vi "TSPopup.Monitor Events.vi"(9 "Debug":bool, 10 "Unregister\nAll Events":bool=TRUE, 11 "TSPopup":refnum<class "TSPopup.lvclass">) -> ()   [LabVIEW 2016, in "TSPopup.lvlib" / "TSPopup.lvclass"]
doc: "Background process that monitors appropriate events when a popup is shown. Sends feedback when popup is complete.\n\nType Sensitive Popup \nCopyright © 2007, J. David Saunders\nAll rights reserved."
uses:
  <userlib>/TSPopup/TSPopup.lvclass
  <userlib>/TSPopup/TSPopup.lvclass/TSPopup.ctl
  <userlib>/TSPopup/Private/TSPopup.Event Enum.ctl
  <userlib>/TSPopup/Private/TSPopup.Popup Results.ctl
  <vilib>/event_ctls.llb/eventvkey.ctl
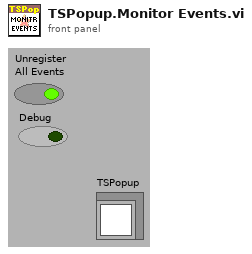
[diagram p1: front panel]
types:
  T1 = enum32{"Invalid", "Standard", "Closed", "Hidden", "Minimized", "Maximized"}
  T2 = typedef "TSPopup.lvlib/TSPopup.lvclass/TSPopup.Event Enum.ctl" = enum16{"Nothing", "Enter Key Accept", "Escape Key Cancel", "Mouse Outside Accept", "Mouse Outside Cancel", "Mouse Move Accept", "Mouse Move Cancel", "Mouse Leave Cancel", "Value Change Accept", "Lose Focus Cancel", "Cancel Button", "Accept Button"}
  T3 = typedef "TSPopup.lvlib/TSPopup.lvclass/TSPopup.Popup Results.ctl" = cluster{"Valid?":bool, "Value Changed?":bool, "Popup Value":variant, "Call Data":variant}
  T4 = typedef "eventvkey.ctl" = enum16{"ASCII", "Enter", "Return", "Shift", "Ctrl", "Alt", "Cmd", "Opt", "Caps", "NumLock", "Clear", "Break", "Up", "Down", "Left", "Right", "Insert", "Delete", "Home", "End", "PageUp", "PageDown", "Escape", "Help", "Pause", "ScrollLock", "F1", "F2", "F3", "F4", "F5", "F6", "F7", "F8", "F9", "F10", "F11", "F12", "F13", "F14", "F15", "F16", "F17", "F18", "F19", "F20", "F21", "F22", "F23", "F24", "Play", "VolumeUp", "VolumeDown", "Mute", "Two Byte Char"}
  T5 = enum32{"Bad", "Idle", "Run top level", "Running"}
  T6 = typedef "TSPopup.lvlib/TSPopup.lvclass/TSPopup.Popup Call Parameters.ctl" = cluster{"Prop Type":T7, "Initial Value":variant, "Caption Strings":string[], "Ring Strings":string[], "Cell Rect":cluster{"left":i16, "top":i16, "right":i16, "bottom":i16}, "Mouse Coords":cluster{"x":i16, "y":i16}, "Call Data":variant}
  T7 = typedef "TSPopup.lvlib/TSPopup.lvclass/TSPopup.Data Type.ctl" = enum16{"Unkown", "NO POPUP", "String", "Integer", "Float", "Color", "Boolean", "Ring", "Captioned String", "Captioned Integer", "Button Color", "2 Int Cluster", "4 Int Cluster", "check"}
  T8 = typedef "LVPoint32TypeDef.ctl" = cluster{"Horizontal":i32, "Vertical":i32}
  T9 = typedef "LVRectTypeDef.ctl" = cluster{"Left":i16, "Top":i16, "Right":i16, "Bottom":i16}
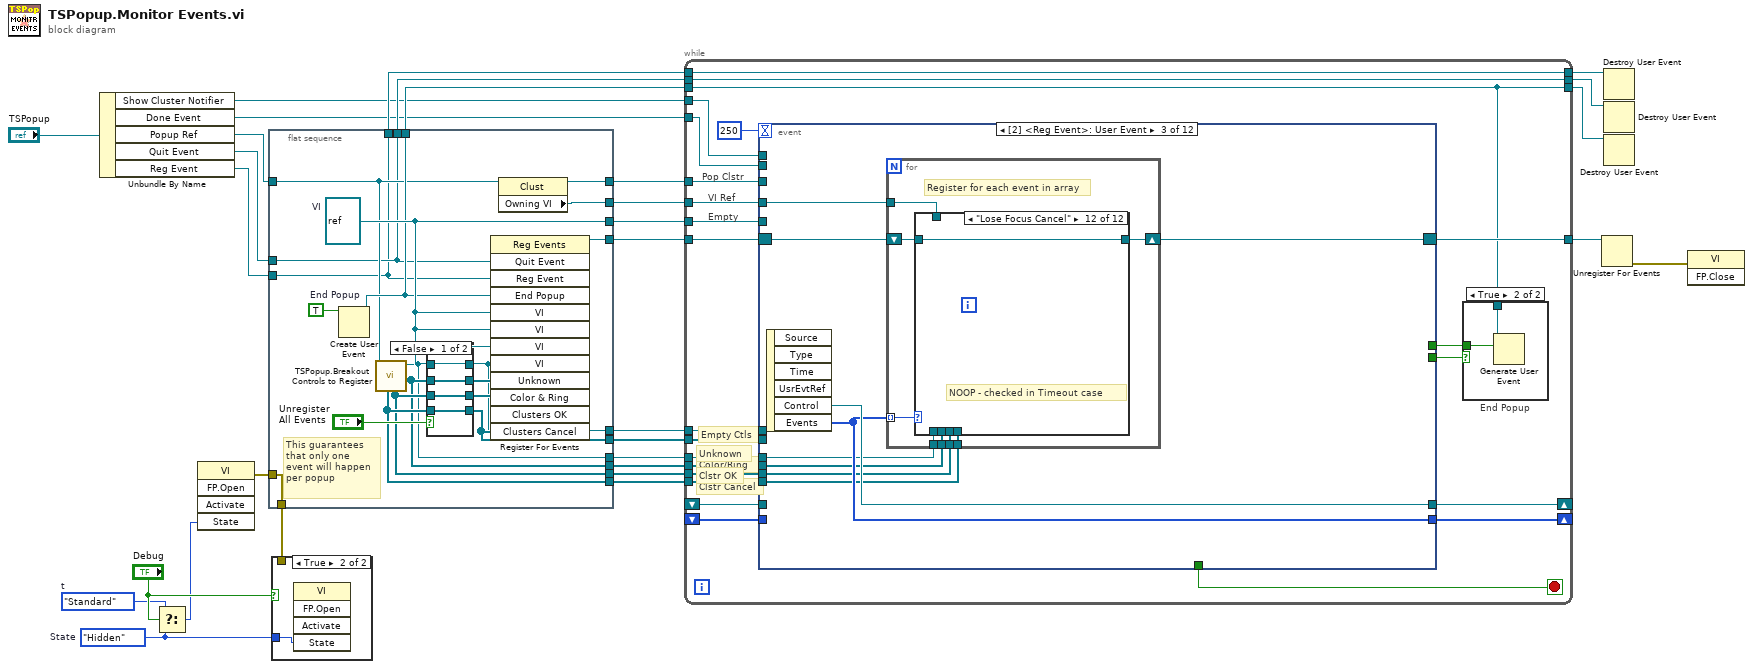
[diagram p0: block diagram]
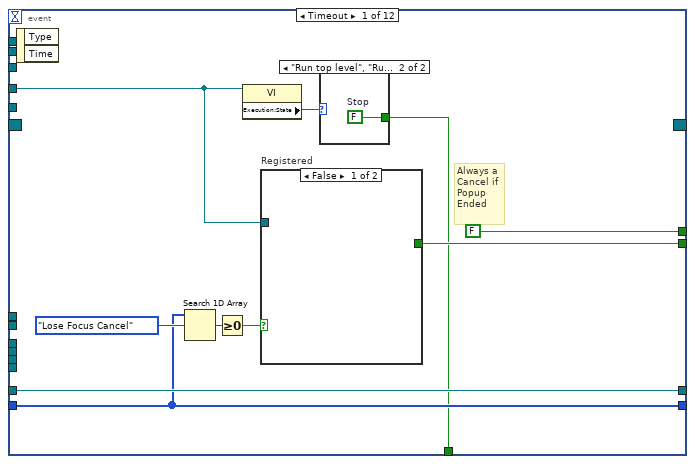
[diagram p5: hidden frame]
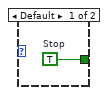
[diagram p6: hidden frame]
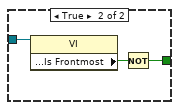
[diagram p7: hidden frame]
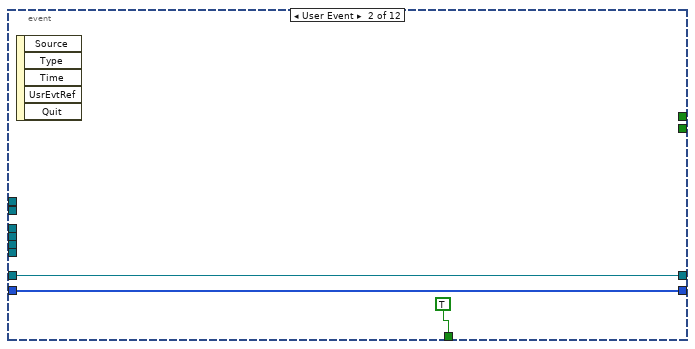
[diagram p8: hidden frame]
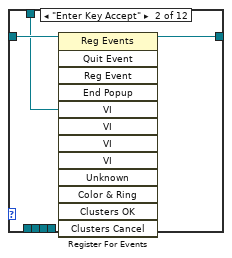
[diagram p10: hidden frame]
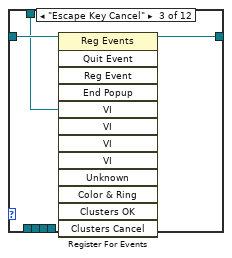
[diagram p11: hidden frame]
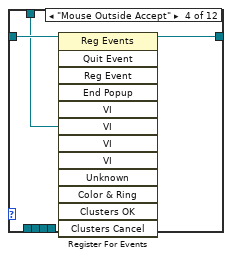
[diagram p12: hidden frame]
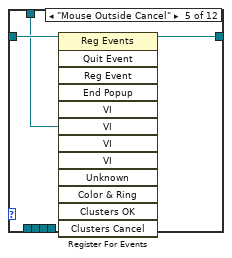
[diagram p13: hidden frame]
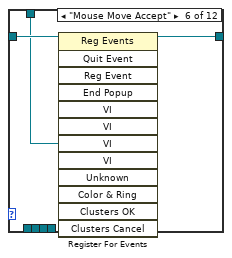
[diagram p14: hidden frame]
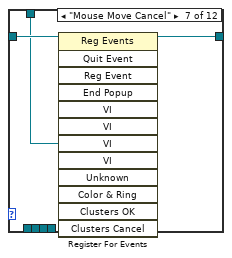
[diagram p15: hidden frame]
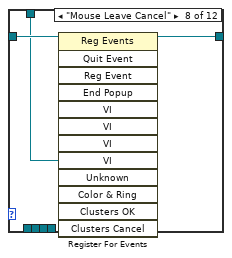
[diagram p16: hidden frame]
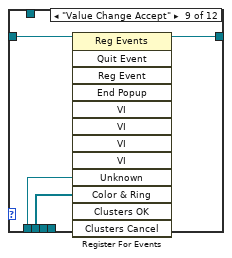
[diagram p17: hidden frame]
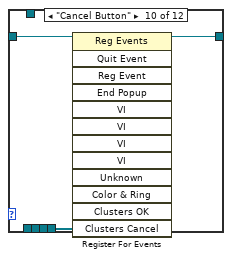
[diagram p18: hidden frame]
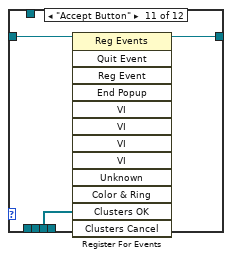
[diagram p19: hidden frame]
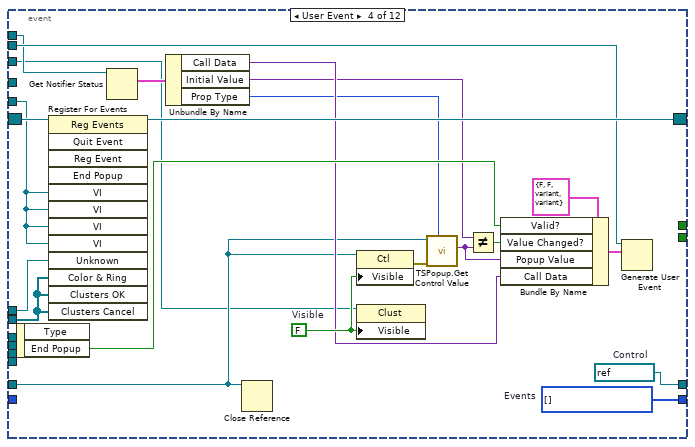
[diagram p20: hidden frame]
diagram:
  w11 = T1."Standard"  # t
  w9 = T1."Hidden"  # State
  n1 = Unbundle By Name("TSPopup") -> ("Show Cluster Notifier"=w2:refnum<notifier>, "Done Event"=w1:refnum<user-event>, "Popup Ref"=w5:refnum<vi>, "Quit Event"=w4:refnum<user-event>, "Reg Event"=w3:refnum<user-event>)
  n2 = Select(t=w11, s="Debug", f=w9) -> (s? t:f=w10:T1)
  n3 = invoke class="VI" method="FP.Open"("State"=w10) -> (error out=w7:errorcluster)  [unwired: 4 in, 4 out]
  n4 = flat-sequence {
    tunnel: [w49] -> w30
    tunnel: [w48] -> w28
    tunnel: [w47] -> w27
    tunnel: [w46] -> w26
    tunnel: [w32] -> w23
    tunnel: [w31] -> w22
    tunnel: [w44] -> w21
    tunnel: [w40] -> w18
    tunnel: [w39] -> w17
    tunnel: [w38] -> w16
    tunnel: [w37] -> w15
    tunnel: [w36] -> w14
    tunnel: [w35] -> w13
    tunnel: w7 -> [w34]
    tunnel: [w34] -> w6
    tunnel: w5 -> [w33]
    tunnel: w4 -> [w32]
    tunnel: w3 -> [w31]
    frame #0 {
      w45 = TRUE  # End Popup
      w46 = refnum<vi> refnum  # VI
      # "This guarantees\nthat only one\nevent will happen\nper popup"
      n5 = Create User Event(user event datatype=w45) -> (user event=w44:refnum<user-event>)  [unwired: 1 in, 1 out]
      n6 = call <userlib>:"TSPopup.Breakout Controls to Register.vi"("Popup"=w33) -> ("Color & Ring"=w38:refnum<vi>[], "Unknown"=w37:refnum<vi>, "Clusters OK"=w39:refnum<vi>[], "Clusters Cancel"=w40:refnum<vi>[])  [unwired: 7 in]
      n7 = case shown="False" "Unregister\nAll Events" {
        tunnel: [w50 _] -> w36
        tunnel: [w51 _] -> w41
        tunnel: [w52 _] -> w42
        tunnel: [w53 _] -> w35
        tunnel: w37 -> [w53 _]
        tunnel: w38 -> [w52 _]
        tunnel: w39 -> [w51 _]
        tunnel: w40 -> [w50 _]
        frame False {
        }
        frame True {
        }
      }
      n8 = register-events(w32, w31, w44, w46, w46, w46, w46, w35, w42, w41, w36) -> (reference out=w49:refnum<event-registration>)  [unwired: 2 in, 1 out]
      n9 = property class="Clust"(reference=w33) -> (reference out=w47:refnum<vi>, "Owning VI"=w48:refnum<vi>)  [unwired: 1 in, 1 out]
    }
  }
  n10 = case shown="True" "Debug" {
    tunnel: w9 -> [_ w54]
    tunnel: w6 -> [_ _]
    frame False {
    }
    frame True {
      n11 = invoke class="VI" method="FP.Open"("State"=w54) -> ()  [unwired: 4 in, 5 out]
    }
  }
  n12 = while {
    tunnel: w30 -> [w77]
    tunnel: w28 -> [w76]
    tunnel: w26 -> [w75]
    tunnel: [w74] -> w29
    tunnel: w27 -> [w73]
    tunnel: w23 -> [w71]
    tunnel: w22 -> [w70]
    tunnel: [w71] -> w24
    tunnel: [w70] -> w25
    shift-right: [w69] -> _
    shift-left: _ -> [w68]
    shift-right: [w67] -> _
    shift-left: _ -> [w66]
    tunnel: w21 -> [w65]
    tunnel: [w65] -> w20
    tunnel: w18 -> [w62]
    tunnel: w17 -> [w61]
    tunnel: w16 -> [w60]
    tunnel: w15 -> [w59]
    tunnel: w14 -> [w58]
    tunnel: w13 -> [w57]
    tunnel: w2 -> [w55]
    tunnel: w1 -> [w56]
    stop <- w72 stop-if-true
    # "Empty Ctls"
    # "Clstr Cancel"
    # "Clstr OK"
    # "Color/Ring"
    # "Unknown"
    # "Pop Clstr"
    # "VI Ref"
    # "Empty"
    n13 = event shown="[2] <Reg Event>: User Event" {
      selector: w77 -> [_ _ w106 w168 _ _ _ _ _ _ _ _]
      dyn-events: [_ _ w104 w166 _ _ _ _ _ _ _ _] -> w74
      timeout: 250 -> [_ _ _ _ _ _ _ _ _ _ _ _]
      tunnel: w76 -> [w83 _ w103 _ _ _ _ _ _ _ _ _]
      tunnel: w75 -> [_ _ _ w167 _ _ _ _ _ _ _ _]
      tunnel: w73 -> [_ _ _ w149 _ _ _ _ _ _ _ _]
      tunnel: [w81 TRUE _ _ _ _ _ _ _ _ _ _] -> w72
      tunnel: [w87 w97 w105 w170 w173 w192 w198 w206 w210 w214 w218 w222] -> w69
      tunnel: w68 -> [w87 w97 _ _ w173 w192 w198 w206 w210 w214 w218 w222]
      tunnel: [w90 w96 w107 w169 w182 w196 w202 w205 w209 w213 w217 w221] -> w67
      tunnel: w66 -> [w90 w96 _ w150 w182 w196 w202 w205 w209 w213 w217 w221]
      tunnel: [w85 _ _ _ w175 w189 TRUE TRUE TRUE TRUE TRUE TRUE] -> w64
      tunnel: [FALSE _ _ _ w174 w188 w197 FALSE FALSE TRUE TRUE FALSE] -> w63
      tunnel: w62 -> [_ _ w99 _ _ _ _ _ _ _ _ _]
      tunnel: w61 -> [_ _ w100 _ _ _ _ _ _ _ _ _]
      tunnel: w60 -> [_ _ w101 _ _ _ _ _ _ _ _ _]
      tunnel: w59 -> [_ _ w102 _ _ _ _ _ _ _ _ _]
      tunnel: w58 -> [_ _ _ w165 _ _ _ _ _ _ _ _]
      tunnel: w57 -> [_ _ _ w164 _ _ _ _ _ _ _ _]
      tunnel: w56 -> [_ _ _ w156 _ _ _ _ _ _ _ _]
      tunnel: w55 -> [_ _ _ w155 _ _ _ _ _ _ _ _]
      event Timeout {
        # "Always a\nCancel if\nPopup\nEnded"
        n14 = event-data() -> ()  [unwired: 1 in, 2 out]
        n15 = Search 1D Array(1D array=w87, element=TSPopup.Event_Enum."Lose Focus Cancel" ("Registered Events")) -> (index of element=w89:i32)  [unwired: 1 in]
        n16 = Greater Or Equal To 0?(x=w89) -> (x >= 0?=w86:bool)
        n17 = property class="VI"(reference=w83) -> ("Execution:State"=w82:T5)  [unwired: 1 in, 2 out]
        n18 = case "Registered" shown="False" w86 {
          tunnel: w83 -> [_ w93]
          tunnel: [_ w94] -> w85
          frame False {
          }
          frame True {
            n19 = property class="VI"(reference=w93) -> ("Front Panel Window:Is Frontmost"=w95:bool)  [unwired: 1 in, 2 out]
            n20 = Not(x=w95) -> (.not. x?=w94:bool)
          }
        }
        n21 = case shown="\"Run top level\", \"Running\"" w82 {
          tunnel: [w91 w92] -> w81
          frame Default {
            w91 = TRUE  # Stop
          }
          frame "Run top level", "Running" {
            w92 = FALSE  # Stop
          }
        }
      }
      event User Event {
        n22 = event-data() -> ()  [unwired: 1 in, 5 out]
      }
      event User Event {
        n23 = event-data() -> ("Control"=w107:refnum<vi>, "Events"=w105:T2[])  [unwired: 1 in, 4 out]
        n24 = for {
          shift-right: [w113] -> w104
          shift-left: w106 -> [w114]
          tunnel: w105 -> [w115] mode=indexing
          tunnel: w103 -> [w112]
          tunnel: w102 -> [w108]
          tunnel: w101 -> [w111]
          tunnel: w100 -> [w109]
          tunnel: w99 -> [w110]
          # "Register for each event in array"
          n25 = case shown="\"Lose Focus Cancel\"" w115 {
            tunnel: w114 -> [w116 w119 w121 w125 w128 w131 w134 w137 w141 w144 w147 w148]
            tunnel: [w116 w118 w122 w124 w127 w130 w133 w136 w140 w143 w146 w148] -> w113
            tunnel: w112 -> [_ w117 w120 w123 w126 w129 w132 w135 _ _ _ _]
            tunnel: w111 -> [_ _ _ _ _ _ _ _ w139 _ _ _]
            tunnel: w110 -> [_ _ _ _ _ _ _ _ _ w142 _ _]
            tunnel: w109 -> [_ _ _ _ _ _ _ _ _ _ w145 _]
            tunnel: w108 -> [_ _ _ _ _ _ _ _ w138 _ _ _]
            frame "Nothing" {
              # "Nothing to register, this\nis default enum value"
            }
            frame "Enter Key Accept" {
              n26 = register-events(reference=w119, w117) -> (reference out=w118:refnum<event-registration>)  [unwired: 11 in, 1 out]
            }
            frame "Escape Key Cancel" {
              n27 = register-events(reference=w121, w120) -> (reference out=w122:refnum<event-registration>)  [unwired: 11 in, 1 out]
            }
            frame "Mouse Outside Accept" {
              n28 = register-events(reference=w125, w123) -> (reference out=w124:refnum<event-registration>)  [unwired: 11 in, 1 out]
            }
            frame "Mouse Outside Cancel" {
              n29 = register-events(reference=w128, w126) -> (reference out=w127:refnum<event-registration>)  [unwired: 11 in, 1 out]
            }
            frame "Mouse Move Accept" {
              n30 = register-events(reference=w131, w129) -> (reference out=w130:refnum<event-registration>)  [unwired: 11 in, 1 out]
            }
            frame "Mouse Move Cancel" {
              n31 = register-events(reference=w134, w132) -> (reference out=w133:refnum<event-registration>)  [unwired: 11 in, 1 out]
            }
            frame "Mouse Leave Cancel" {
              n32 = register-events(reference=w137, w135) -> (reference out=w136:refnum<event-registration>)  [unwired: 11 in, 1 out]
            }
            frame "Value Change Accept" {
              n33 = register-events(reference=w141, w138, w139) -> (reference out=w140:refnum<event-registration>)  [unwired: 10 in, 1 out]
            }
            frame "Cancel Button" {
              n34 = register-events(reference=w144, w142) -> (reference out=w143:refnum<event-registration>)  [unwired: 11 in, 1 out]
            }
            frame "Accept Button" {
              n35 = register-events(reference=w147, w145) -> (reference out=w146:refnum<event-registration>)  [unwired: 11 in, 1 out]
            }
            frame "Lose Focus Cancel" {
              # "NOOP - checked in Timeout case"
            }
          }
        }
      }
      event User Event {
        w158 = FALSE  # Visible
        w169 = refnum<vi> refnum  # Control
        w170 = T2[] [] items=["Nothing", "Enter Key Accept", "Escape Key Cancel", "Mouse Outside Accept", "Mouse Outside Cancel", "Mouse Move Accept", "Mouse Move Cancel", "Mouse Leave Cancel", "Value Change Accept", "Lose Focus Cancel", "Cancel Button", "Accept Button"]  # Events
        n36 = event-data() -> ("End Popup"=w157:bool)  [unwired: 1 in, 1 out]
        n37 = register-events(reference=w168, w167, w167, w167, w167, w164, w165, w165, w165) -> (reference out=w166:refnum<event-registration>)  [unwired: 4 in, 1 out]
        n38 = Get Notifier Status(notifier=w155) -> (current notification=w154:T6)  [unwired: 1 in, 4 out]
        n39 = Unbundle By Name(w154) -> ("Call Data"=w153:variant, "Initial Value"=w152:variant, "Prop Type"=w151:T7)
        n40 = Close Reference(reference=w150) -> ()  [unwired: 1 in, 1 out]
        n41 = property on="Property Node" class="Ctl"(reference=w150, "Visible"=w158) -> (error out=w159:errorcluster)  [unwired: 1 in, 1 out]
        n42 = property class="Clust"(reference=w149, "Visible"=w158) -> ()  [unwired: 1 in, 2 out]
        n43 = call <userlib>:"TSPopup.Get Control Value.vi"("Prop Type"=w151, "error in (no error)"=w159, "Control"=w150) -> ("Value"=w161:variant)  [unwired: 6 in, 2 out]
        n44 = Not Equal?(x=w152, y=w161) -> (x != y?=w160:bool)
        n45 = Bundle By Name(cluster=T3 {"Valid?"=FALSE, "Value Changed?"=FALSE, "Popup Value"=variant, "Call Data"=variant} ("Popup Results (type only)"), "Valid?"=w157, "Value Changed?"=w160, "Popup Value"=w161, "Call Data"=w153) -> (w163:T3)
        n46 = Generate User Event(user event=w156, event data cluster=w163) -> ()  [unwired: 2 in, 2 out]
      }
      event Key Down? {
        w180 = TSPopup.Event_Enum."Escape Key Cancel"  # element
        # "Enter = Accept Popup"
        # "Registered Key Pressed"
        # "Check that key is \nRegistered and Pressed"
        # "Verify that\nkey was also\nregistered"
        # "Check if correct\nkey was pressed"
        n47 = event-data() -> ("VKey"=w171:T4)  [unwired: 1 in, 8 out]
        n48 = call <vilib>:"compatReturnToEnter.vi"("VKey"=w171) -> ("VKey"=w172:T4)
        n49 = Search 1D Array(1D array=w173, element=w180) -> (index of element=w181:i32)  [unwired: 1 in]
        n50 = Search 1D Array(1D array=w173, element=TSPopup.Event_Enum."Enter Key Accept") -> (index of element=w177:i32)  [unwired: 1 in]
        n51 = Greater Or Equal To 0?(x=w181) -> (x >= 0?=w179:bool)
        n52 = Greater Or Equal To 0?(x=w177) -> (x >= 0?=w176:bool)
        n53 = Equal?(x=eventvkey."Escape" ("VKey"), y=w172) -> (x = y?=w185:bool)
        n54 = Equal?(x=w172, y=eventvkey."Enter") -> (x = y?=w183:bool)
        n55 = And(x=w185, y=w179) -> (x .and. y?=w184:bool)
        n56 = And(x=w176, y=w183) -> (x .and. y?=w174:bool)
        n57 = Or(x=w184, y=w174) -> (x .or. y?=w175:bool)
        n58 = event-data("Discard?"=w175) -> ()  [unwired: 4 in, 1 out]
      }
      event Mouse Down? {
        # "Not in Control"
        n59 = event-data() -> ("Coords"=w195:T8)  [unwired: 1 in, 7 out]
        n60 = property class="Ctl"(reference=w196) -> ("Total Bounds Rect"=w194:T9)  [unwired: 1 in, 2 out]
        n61 = call <vilib>:"PointInRect.vi"("rect"=w194, "point"=w195) -> ("pt in rect"=w190:bool)
        n62 = Not(x=w190) -> (.not. x?=w189:bool)
        n63 = Search 1D Array(1D array=w192, element=TSPopup.Event_Enum."Mouse Outside Accept" ("Registered Events")) -> (index of element=w193:i32)  [unwired: 1 in]
        n64 = Greater Or Equal To 0?(x=w193) -> (x >= 0?=w188:bool)
        n65 = event-data("Discard?"=w189) -> ()  [unwired: 4 in, 1 out]
      }
      event Mouse Move {
        # "Used for Rings to capture when the selection doesn't change\nand for both rings and colorboxes when Escape is pressed \n(not captured with Key Press event)"
        n66 = event-data() -> ()  [unwired: 1 in, 5 out]
        n67 = Search 1D Array(1D array=w198, element=TSPopup.Event_Enum."Mouse Move Accept" ("Registered Events")) -> (index of element=w200:i32)  [unwired: 1 in]
        n68 = Greater Or Equal To 0?(x=w200) -> (x >= 0?=w197:bool)
      }
      event Mouse Leave {
        # "Mouse Leave is (currently) always registered as a cancel.\nThis is used for Colors and Rings to capture when the Escape key is\npressed when the mouse is outside the window."
        n69 = event-data() -> ()  [unwired: 1 in, 4 out]
      }
      event Value Change {
        # "If Data Type is unknown, a Button is displayed.\n\nReturn Canceled after button is pressed"
        n70 = event-data() -> ()  [unwired: 1 in, 6 out]
      }
      event Value Change {
        # "Value Change for Color Box and Ring is registered\n\nThe value changes for other data types are ignored -- their\nevents are captured via mouse or keyboard events."
        n71 = event-data() -> ()  [unwired: 1 in, 6 out]
      }
      event Value Change {
        n72 = event-data() -> ()  [unwired: 1 in, 6 out]
      }
      event Value Change {
        n73 = event-data() -> ()  [unwired: 1 in, 6 out]
      }
    }
    n74 = case "End Popup" shown="True" w64 {
      tunnel: w65 -> [_ w80]
      tunnel: w63 -> [_ w79]
      frame False {
      }
      frame True {
        n75 = Generate User Event(user event=w80, event data cluster=w79) -> ()  [unwired: 2 in, 2 out]
      }
    }
  }
  n76 = Unregister For Events(event registration refnum=w29) -> (error out=w19:errorcluster)  [unwired: 1 in]
  n77 = Destroy User Event(user event=w25) -> ()  [unwired: 1 in, 1 out]
  n78 = Destroy User Event(user event=w24) -> ()  [unwired: 1 in, 1 out]
  n79 = Destroy User Event(user event=w20) -> ()  [unwired: 1 in, 1 out]
  n80 = invoke class="VI" method="FP.Close"(error in=w19) -> ()  [unwired: 2 in, 3 out]
